vi "CleanupDAQTasks.vi"(8 "error in (no error)":errorcluster, 11 "Queue in":refnum<queue>) -> (0 "error out":errorcluster, 3 "Queue out":refnum<queue>)   [LabVIEW 2014, in "GageLv.lvlib"]
uses:
  <instrlib>/GageLv_uic/GageLv.lvlib
  <instrlib>/GenericDAQ/VI/GenericDAQ_Ctrl_Queue.ctl
  <instrlib>/GenericDAQ/VI/GenericDAQ_State.ctl
  <instrlib>/GenericDAQ/GenericDAQ.lvlib
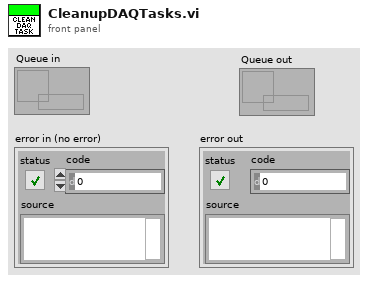
[diagram p1: front panel]
types:
  T1 = typedef "GenericDAQ.lvlib/GenericDAQ_Ctrl_Queue.ctl" = cluster{"GenericDAQ State":T2, "Variant":variant}
  T2 = typedef "GenericDAQ.lvlib/GenericDAQ_State.ctl" = enum16{"Enumerate", "Open", "Close", "CloseAll", "Reset", "Quit", "==Settings==", "SetAcquisition_", "SetChannels_", "SetTrigger_", "SetAnalogTrigDetector_", "SetAll_AcquChTrig_", "fConfigurate", "fStart", "GetStatus", "_WaitForDone/Idle", "_GetData", "GetAcquisition", "GetChannels", "GetTrigger", "GetAll_AcquChTrig", "==Messaging==", "_PushDataOut", "GetStat_", "GetConfig_", "==ModeSetup==", "SetSignalBuffer_", "SetMode_", "SetSecondaryDataRef._", "SetDynamicBuffer_", "==AnalogOut==", "GetChannelCount_AO", "fStart_AO", "SetChEnable_AO", "SetConfig_AO", "SetFuncData_AO", "SetOffset_AO_", "SetMasterNode_AO", "SetStates_AO", "SetSymetry_AO", "SetTriggerSource_AO", "==Trigger==", "ManualTrigger", "===Sync===", "LineStart", "LineEnd", "FrameStart", "FrameEnd", "EOL_PassThrough", "SOL_PassThrough"}
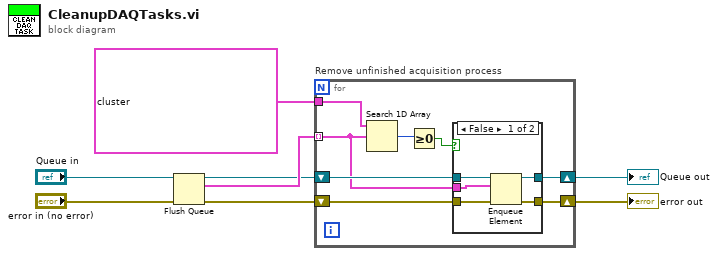
[diagram p0: block diagram]
diagram:
  n1 = Flush Queue(queue="Queue in", error in (no error)="error in (no error)") -> (queue out=w2:refnum<queue>, remaining elements=w4:T1[], error out=w3:errorcluster)
  n2 = for "Remove unfinished acquisition process" {
    shift-right: [w15] -> w1
    shift-left: w2 -> [w16]
    shift-right: [w13] -> w6
    shift-left: w3 -> [w14]
    tunnel: w4 -> [w9] mode=indexing
    tunnel: T1[] [{"GenericDAQ State"=enum."_WaitForDone/Idle", "Variant"=variant}, {"GenericDAQ State"=enum."_GetData", "Variant"=variant}, {"GenericDAQ State"=enum."_PushDataOut", "Variant"=variant}] ("remaining elements") -> [w12]
    n3 = Search 1D Array(1D array=w12, element=w9) -> (index of element=w11:i32)  [unwired: 1 in]
    n4 = Greater Or Equal To 0?(x=w11) -> (x >= 0?=w10:bool)
    n5 = case shown="False" w10 {
      tunnel: w16 -> [w21 w23]
      tunnel: [w20 w23] -> w15
      tunnel: w14 -> [w19 w22]
      tunnel: [w18 w22] -> w13
      tunnel: w9 -> [w17 _]
      frame False {
        n6 = Enqueue Element(queue=w21, element=w17, error in (no error)=w19) -> (queue out=w20:refnum<queue>, error out=w18:errorcluster)  [unwired: 1 in, 1 out]
      }
      frame True {
      }
    }
  }
  "error out" <- w6
  "Queue out" <- w1
